vi "Get IP Address.vi"(8 "error in (no error)":errorcluster, 11 "Default Address":string="0.0.0.0") -> (0 "error out":errorcluster, 3 "IPv4 Address":string)   [LabVIEW 2021, in "CIFCoreCommon.lvlib"]
uses:
  CIFCoreCommon.lvlib
  <vilib>/CIF Foundation/CIF Utilities/Networking/Networking_CIF_U.lvlib
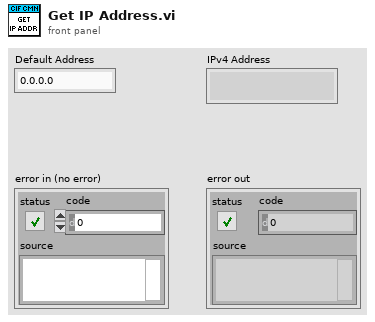
[diagram p1: front panel]
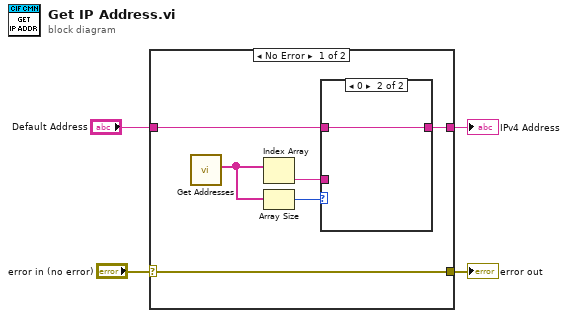
[diagram p0: block diagram]
diagram:
  n1 = case shown="No Error" "error in (no error)" {
    selector: "error in (no error)" -> [w5 w14]
    tunnel: [w10 w13] -> w4
    tunnel: "Default Address" -> [w9 w13]
    tunnel: [w5 w14] -> w1
    frame No Error {
      n2 = call <vilib>:"Get Addresses.vi"() -> ("Addresses"=w7:string[])  [unwired: 10 in, 1 out]
      n3 = Index Array(array=w7) -> (element=w6:string)  [unwired: 1 in]
      n4 = Array Size(array=w7) -> (size(s)=w8:i32)
      n5 = case shown="0" w8 {
        tunnel: w6 -> [w11 _]
        tunnel: [w11 w12] -> w10
        tunnel: w9 -> [_ w12]
        frame 1, Default {
        }
        frame 0 {
        }
      }
    }
    frame Error {
    }
  }
  "error out" <- w1
  "IPv4 Address" <- w4
